vi "test Dequeue Timeout.vi"(8 "error in (no error)":errorcluster, 11 "TestCase in":refnum<class "Message Queue Test Case.lvclass">) -> (0 "error out":errorcluster, 3 "TestCase out":refnum<class "Message Queue Test Case.lvclass">)   [LabVIEW 2017, in "Message Queue Test Case.lvclass"]
uses:
  Message Queue Test Case.lvclass
  Message/Abstract Message/Abstract Message.lvclass
  Message Queue Test Case.lvclass/Message Queue Test Case.ctl
  Message Queue/Abstract Message Queue/Abstract Message Queue.lvclass
  <vilib>/addons/_JKI Toolkits/VI Tester/TestCase.llb/TestCase.lvclass
  C:/Program Files (x86)/National Instruments/LabVIEW 2017/vi.lib/addons/_JKI Toolkits/VI Tester/TestCase.llb/TestCase.lvclass
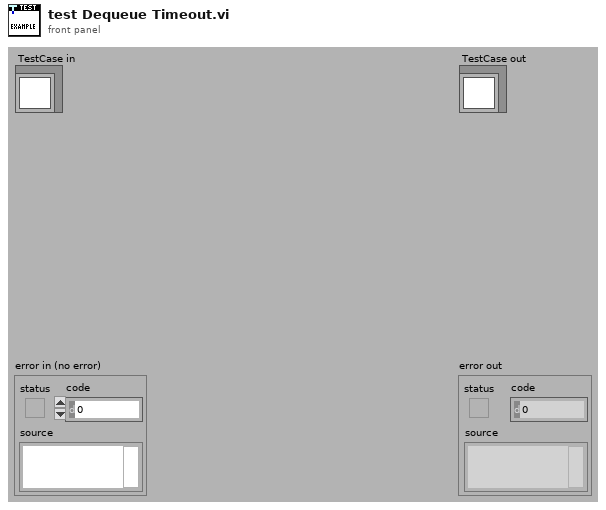
[diagram p1: front panel]
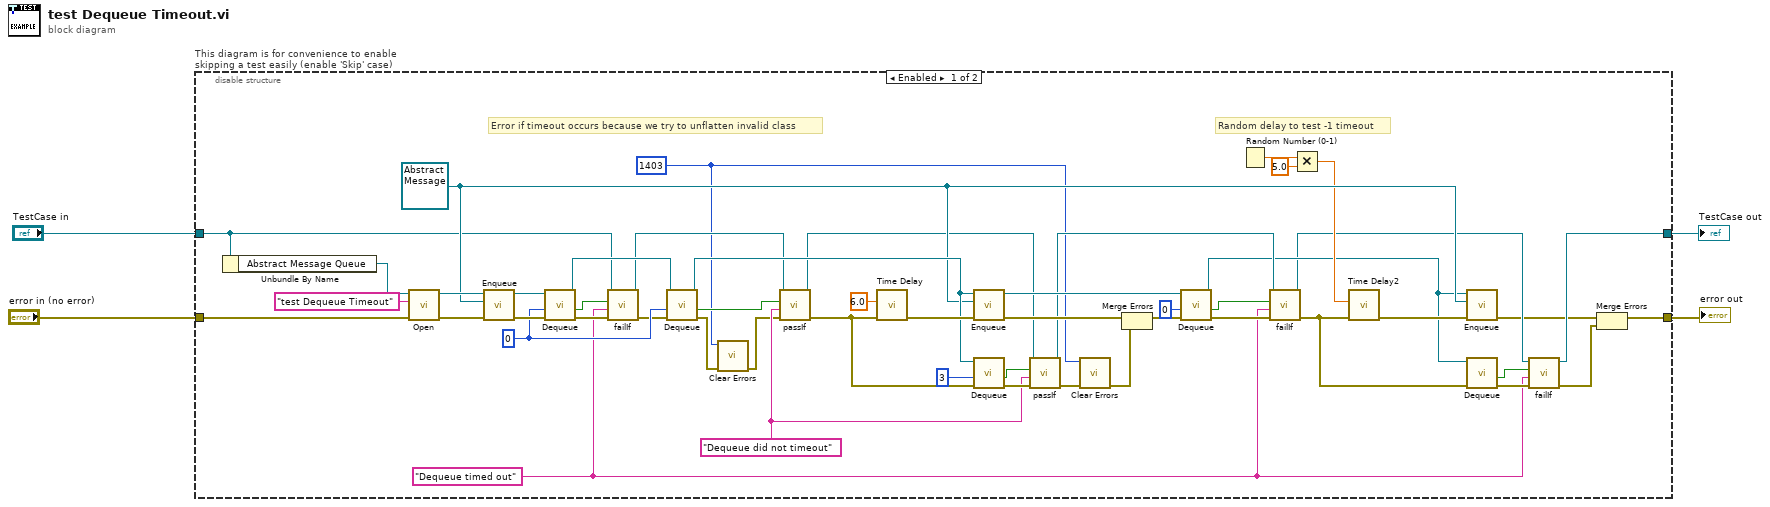
[diagram p0: block diagram]
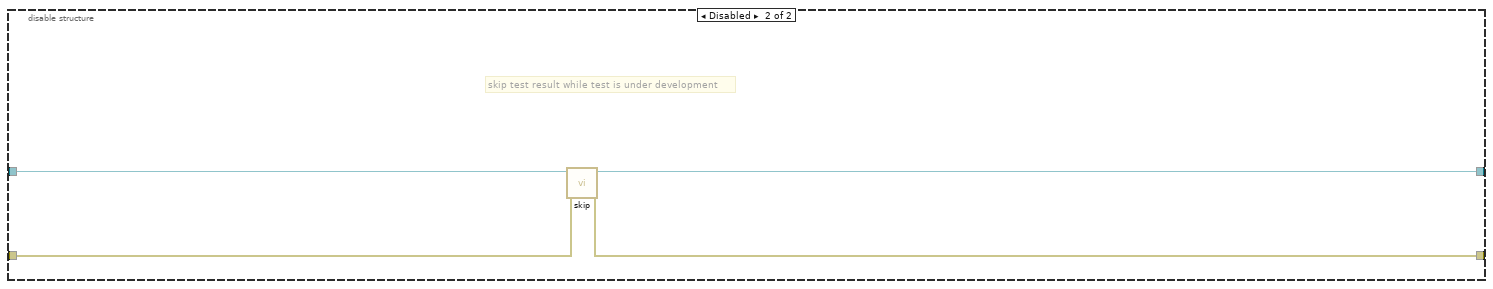
[diagram p2: hidden frame]
diagram:
  n1 = disable-structure "This diagram is for convenience to enable skipping a test easily (enable 'Skip' case)" shown="Enabled" {
    disable-tunnel: "TestCase in" -> [w31 w59]
    disable-tunnel: [w14 w57] -> w1
    disable-tunnel: [w11 w58] -> w3
    disable-tunnel: "error in (no error)" -> [w55 w56]
    frame Enabled {
      w5 = 1403 ("specific error code to clear (0: all)")
      w16 = "Dequeue timed out" ("message (\"\")")
      w40 = "Dequeue did not timeout" ("message (\"\")")
      w47 = 0 ("timeout in ms (-1)")
      w33 = refnum<class "Abstract Message.lvclass"> refnum ("Message in")
      # "Random delay to test -1 timeout"
      # "Error if timeout occurs because we try to unflatten invalid class"
      n2 = Unbundle By Name(w31) -> ("Abstract Message Queue"=w54:refnum<class "Abstract Message Queue.lvclass">)
      n3 = call-dynamic "Open.vi"("error in (no error)"=w55, "name (unnamed)"="test Dequeue Timeout", "Abstract Message Queue in"=w54) -> ("error out"=w52:errorcluster, "Abstract Message Queue out"=w51:refnum<class "Abstract Message Queue.lvclass">)  [unwired: 7 in]
      n4 = call-dynamic "Enqueue.vi"("error in (no error)"=w52, "Message in"=w33, "Abstract Message Queue in"=w51) -> ("error out"=w50:errorcluster, "Abstract Message Queue out"=w49:refnum<class "Abstract Message Queue.lvclass">)  [unwired: 7 in]
      n5 = call-dynamic "Dequeue.vi"("error in (no error)"=w50, "timeout in ms (-1)"=w47, "Abstract Message Queue in"=w49) -> ("error out"=w32:errorcluster, "timed out?"=w21:bool, "Abstract Message Queue out"=w48:refnum<class "Abstract Message Queue.lvclass">)  [unwired: 5 in, 1 out]
      n6 = call-dynamic "failIf.vi"("error in (no error)"=w32, "message (\"\")"=w16, "fail"=w21, "TestCase in"=w31) -> ("error out"=w10:errorcluster, "TestCase out"=w30:refnum<class "Message Queue Test Case.lvclass">)  [unwired: 6 in]
      n7 = call-dynamic "Dequeue.vi"("error in (no error)"=w10, "timeout in ms (-1)"=w47, "Abstract Message Queue in"=w48) -> ("error out"=w9:errorcluster, "timed out?"=w46:bool, "Abstract Message Queue out"=w39:refnum<class "Abstract Message Queue.lvclass">)  [unwired: 5 in, 1 out]
      n8 = call <vilib>:"Clear Errors.vi"("error in (no error)"=w9, "specific error code to clear (0: all)"=w5) -> ("error out"=w8:errorcluster)  [unwired: 4 in, 1 out]
      n9 = call-dynamic "passIf.vi"("error in (no error)"=w8, "message (\"\")"=w40, "pass"=w46, "TestCase in"=w30) -> ("error out"=w44:errorcluster, "TestCase out"=w27:refnum<class "Message Queue Test Case.lvclass">)  [unwired: 6 in]
      n10 = call "Time Delay"("error in (no error)"=w44, "Delay Time (s)"=6.0) -> ("error out"=w43:errorcluster)  [unwired: 9 in]
      n11 = call-dynamic "Enqueue.vi"("error in (no error)"=w43, "Message in"=w33, "Abstract Message Queue in"=w39) -> ("error out"=w37:errorcluster, "Abstract Message Queue out"=w35:refnum<class "Abstract Message Queue.lvclass">)  [unwired: 7 in]
      n12 = call-dynamic "Dequeue.vi"("error in (no error)"=w44, "timeout in ms (-1)"=3, "Abstract Message Queue in"=w39) -> ("error out"=w42:errorcluster, "timed out?"=w41:bool)  [unwired: 5 in, 2 out]
      n13 = call-dynamic "passIf.vi"("error in (no error)"=w42, "message (\"\")"=w40, "pass"=w41, "TestCase in"=w27) -> ("error out"=w7:errorcluster, "TestCase out"=w26:refnum<class "Message Queue Test Case.lvclass">)  [unwired: 6 in]
      n14 = call <vilib>:"Clear Errors.vi"("error in (no error)"=w7, "specific error code to clear (0: all)"=w5) -> ("error out"=w6:errorcluster)  [unwired: 4 in, 1 out]
      n15 = Merge Errors(w37, w6) -> (w36:errorcluster)
      n16 = call-dynamic "Dequeue.vi"("error in (no error)"=w36, "timeout in ms (-1)"=0, "Abstract Message Queue in"=w35) -> ("error out"=w28:errorcluster, "timed out?"=w20:bool, "Abstract Message Queue out"=w18:refnum<class "Abstract Message Queue.lvclass">)  [unwired: 5 in, 1 out]
      n17 = Random Number (0-1)() -> (number: 0 to 1=w24:dbl)
      n18 = call-dynamic "failIf.vi"("error in (no error)"=w28, "message (\"\")"=w16, "fail"=w20, "TestCase in"=w26) -> ("error out"=w25:errorcluster, "TestCase out"=w15:refnum<class "Message Queue Test Case.lvclass">)  [unwired: 6 in]
      n19 = Multiply(x=w24, y=5.0) -> (x*y=w22:dbl)
      n20 = call "Time Delay2"("error in (no error)"=w25, "Delay Time (s)"=w22) -> ("error out"=w29:errorcluster)  [unwired: 9 in]
      n21 = call-dynamic "Enqueue.vi"("error in (no error)"=w29, "Message in"=w33, "Abstract Message Queue in"=w18) -> ("error out"=w13:errorcluster)  [unwired: 7 in, 1 out]
      n22 = call-dynamic "Dequeue.vi"("error in (no error)"=w25, "Abstract Message Queue in"=w18) -> ("error out"=w19:errorcluster, "timed out?"=w17:bool)  [unwired: 6 in, 2 out]
      n23 = call-dynamic "failIf.vi"("error in (no error)"=w19, "message (\"\")"=w16, "fail"=w17, "TestCase in"=w15) -> ("error out"=w12:errorcluster, "TestCase out"=w14:refnum<class "Message Queue Test Case.lvclass">)  [unwired: 6 in]
      n24 = Merge Errors(w13, w12) -> (w11:errorcluster)
    }
    frame Disabled {
      # "skip test result while test is under development"
      n25 = call <vilib>:"skip.vi"("error in (no error)"=w56, "TestCase in"=w59) -> ("error out"=w58:errorcluster, "TestCase out"=w57:refnum<class "Message Queue Test Case.lvclass">)  [unwired: 8 in]
    }
  }
  "error out" <- w3
  "TestCase out" <- w1
